vi "Write Visible.vi"(5 "Visible":bool, 9 "Scale in":refnum<class "Scale.lvclass">) -> (3 "Scale out":refnum<class "Scale.lvclass">)   [LabVIEW 2014, in "Scale.lvclass"]
uses:
  Scale.lvclass
  Scale.lvclass/Scale.ctl
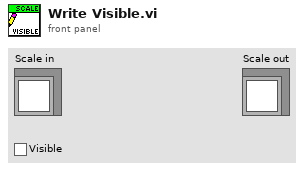
[diagram p1: front panel]
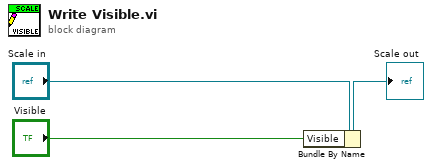
[diagram p0: block diagram]
diagram:
  n1 = Bundle By Name(cluster="Scale in", "Visible"="Visible") -> (→"Scale out":refnum<class "Scale.lvclass">)
